vi "Handle Error.vi"(8 "error in (no error)":errorcluster, 11 "TCP Writer in":refnum<class "TCP Writer.lvclass">) -> (0 "error out":errorcluster, 2 "stop actor?":bool=TRUE, 3 "TCP Writer out":refnum<class "TCP Writer.lvclass">)   [LabVIEW 2018, in "TCP Classes.lvlib" / "TCP Writer.lvclass"]
doc: "(<B>Filename</B>: Actor Framework.lvlib:Actor.lvclass:Handle Error.vi)\n\nDefines how the actor handles an error that occurred while processing a message.\n\nBy default, this method does nothing except stop the actor. This method also treats error code 43 (coming from <B>error in</B>) as a sign that the actor shut down normally. In this situation, the Handle Error method does not return the error on <B>error out</B>, meaning the actor's caller will not receive it. All other error codes will be returned on <B>error out</B>.\n\nA descendant class may override this method to change this behavior."
uses:
  TCP Writer.lvclass
  C:/Program Files (x86)/National Instruments/LabVIEW 2018/vi.lib/ActorFramework/Actor/Actor.lvclass
  <vilib>/ActorFramework/Actor/Actor.lvclass/Actor.ctl
  Actor Nest/Actor Nest Messages/Handle Nested Error Msg/Handle Nested Error Msg.lvclass/Handle Nested Error Msg.ctl
  <vilib>/ActorFramework/Message Enqueuer/Message Enqueuer.lvclass/Message Enqueuer.ctl
  <vilib>/ActorFramework/Message Enqueuer/Enqueue.vi
  Actor Nest/Actor Nest Messages/Handle Nested Error Msg/Handle Nested Error Msg.lvclass
  C:/Program Files (x86)/National Instruments/LabVIEW 2018/vi.lib/ActorFramework/Message/Message.lvclass
  <vilib>/ActorFramework/Message Priority Queue/Priority Enqueue.vi
  Class TCP Connection/TCP Connection.lvclass
  <vilib>/ActorFramework/Actor/Actor.lvclass
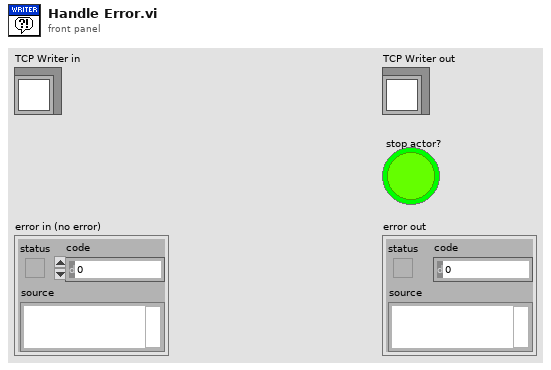
[diagram p1: front panel]
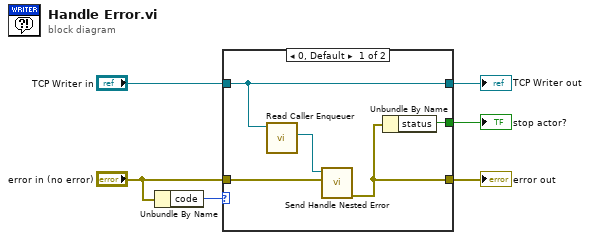
[diagram p0: block diagram]
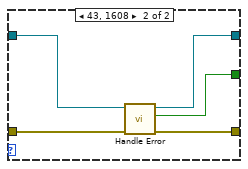
[diagram p2: hidden frame]
diagram:
  n1 = Unbundle By Name("error in (no error)") -> ("code"=w1:i32)
  n2 = case shown="0, Default" w1 {
    tunnel: [w10 w16] -> w6
    tunnel: [w9 w15] -> w5
    tunnel: [w8 w14] -> w4
    tunnel: "error in (no error)" -> [w11 w13]
    tunnel: "TCP Writer in" -> [w8 w12]
    frame 0, Default {
      n3 = call <vilib>:"Read Caller Enqueuer.vi"("Actor"=w8) -> ("Caller Enqueuer"=w7:refnum<class "Message Enqueuer.lvclass">)  [unwired: 10 in]
      n4 = call "Send Handle Nested Error.vi"("Nested Error"=w11, "Message Enqueuer"=w7) -> ("error out"=w10:errorcluster)  [unwired: 8 in, 1 out]
      n5 = Unbundle By Name(w10) -> ("status"=w9:bool)
    }
    frame 43, 1608 {
      n6 = call-parent "Handle Error.vi"("error in (no error)"=w13, "Actor in"=w12) -> ("error out"=w16:errorcluster, "stop actor?"=w15:bool, "Actor out"=w14:refnum<class "TCP Writer.lvclass">)  [unwired: 7 in]
    }
  }
  "TCP Writer out" <- w4
  "error out" <- w6
  "stop actor?" <- w5
